vi "save_mpi_hdf.vi"(3 "System Information cluster":T1, 5 "Subject metadata cluster":T2, 7 "Device Name":tag="DAQ2", 8 "TxRxParams":T3={"sample rate"=1000000.0, "Transmit frequency"=25000.0, "Transmit amplitude"=1.577, "sample rate digital out"=40000.0, "TX cycles"=600, "sample rate DAQ1"=1000000.0, "Receive frequency"=75000.0, "Receive range"=1.0, "TX harmonics"=[50000.0, 75000.0, 100000.0, 125000.0, 150000.0, 175000.0, 200000.0, 225000.0]} {"TX harmonics" format="%#_6p"; "Receive frequency" format="%#_6p"; "sample rate DAQ1" format="%#_6p"; "sample rate digital out" format="%#_6p"; "Transmit frequency" format="%#_6p"; "sample rate" format="%#_6p"}, 9 "image dataset":string, 10 "Path":path, 11 "Cluster in":T4={"Magnitude meas."=[], "Phase meas."=[], "Shift meas."=[], "cw"=TRUE, "projections per image"=0, "ramp-up readouts"=0, "current sense type"="", "Number of pulses per image"=0, "Rotation enabled"=TRUE, "Rotary position"=[], "Baseline magnitude"=0.0, "Baseline phase"=0.0, "Wait readouts"=0, "Shift waveform type"="", "Shift enabled"=TRUE, "Time domain data"=[], "Motor pulse duration"=0.0, "Shift Amp pk"=0.0, "Shift DC offset"=0.0, "Notes"="", "Reconstructed image"=bytes[0], "Rotary encoder type"="", "Image start"=timestamp(0 s since 1904-01-01), "Image stop"=timestamp(0 s since 1904-01-01), "readouts per projection"=0, "Recon enabled"=FALSE, "Bidirectional shift"=FALSE, "Imager mode"="", "Shift delay"=0.0, "Shift frequency"=0.0, "Image time (calc)"=0.0, "Initial encoder position"=0.0, "Recon data"=[], "Trigger line values"=[], "Bed position"=0.0, "Sample image"=bytes[0], "Patch amplitude"=0.0, "Patch frequency"=0.0, "Patch phase"=0.0, "proj mag f2-f9"=[], "proj phase f2-f9"=[], "Tx waveform"=[], "Tx FFT mag"=[], "Tx FFT phase"=[], "Temps"=[]}) -> ()   [LabVIEW 2021]
uses:
  <vilib>/UPVI/lvhdf5/file.llb/LVH5F Operation.ctl
  <vilib>/Utility/miscctls.llb/LVRectTypeDef.ctl
  <vilib>/UPVI/lvhdf5/group.llb/H5G_obj_t.ctl
  <vilib>/UPVI/lvhdf5/dataset.llb/LVH5D Operation.ctl
  <vilib>/UPVI/lvhdf5/attribute.llb/LVH5A Operation.ctl
  <vilib>/UPVI/lvhdf5/identifier.llb/Not an HDF5 Refnum Constant.vi
  <vilib>/UPVI/lvhdf5/utility.llb/Select HDF5 Dialog.vi
  <vilib>/UPVI/lvhdf5/utility.llb/Select HDF5 Dialog (Object Only).vi
  <vilib>/UPVI/lvhdf5/dataset.llb/Simple H5Dwrite (Variant).vi
  <vilib>/UPVI/lvhdf5/common.llb/To HDF5 Ref.vi
  <vilib>/UPVI/lvhdf5/dataset.llb/H5Dclose.vi
  <vilib>/UPVI/lvhdf5/attribute.llb/LVH5 Write Attributes.xnode
  <vilib>/UPVI/lvhdf5/library.llb/HDF5 Ref.ctl
  <vilib>/UPVI/lvhdf5/dataset.llb/Simple H5Dwrite.xnode
  <vilib>/UPVI/lvhdf5/dataset.llb/Write Dataset with Attributes.xnode
  <vilib>/UPVI/lvhdf5/attribute.llb/Cluster to Attribute Array.xnode
  <vilib>/Utility/error.llb/Error Cluster From Error Code.vi
  <vilib>/UPVI/lvhdf5/dataset.llb/OpenCreateReplace Dataset by Element Type.vi
  <vilib>/UPVI/lvhdf5/dataspace.llb/H5Sselect_hyperslab.vi
  <vilib>/UPVI/lvhdf5/dataset.llb/H5Dwrite (Variant).vi
  <vilib>/UPVI/lvhdf5/dataset.llb/H5Dget_space.vi
  <vilib>/UPVI/lvhdf5/attribute.llb/private/LVH5AwriteWDTAttrs.vi
  <vilib>/UPVI/lvhdf5/dataspace.llb/H5Sclose.vi
  <vilib>/UPVI/lvhdf5/utility.llb/Select HDF5 Dialog (File and Object).vi
  <resource>/objmgr/daqmx.rc
  <vilib>/UPVI/lvhdf5/library.llb/HDF5 Ref.lvclass
  <vilib>/Utility/Data Type/Get Type Information.vi
  <vilib>/Utility/Data Type/NI_Data Type.lvlib
  <vilib>/Utility/Data Type/Get Cluster Information.vi
panel:
  in  "OnlineReconPath":path
  out "appended path":path
  out "error out":errorcluster
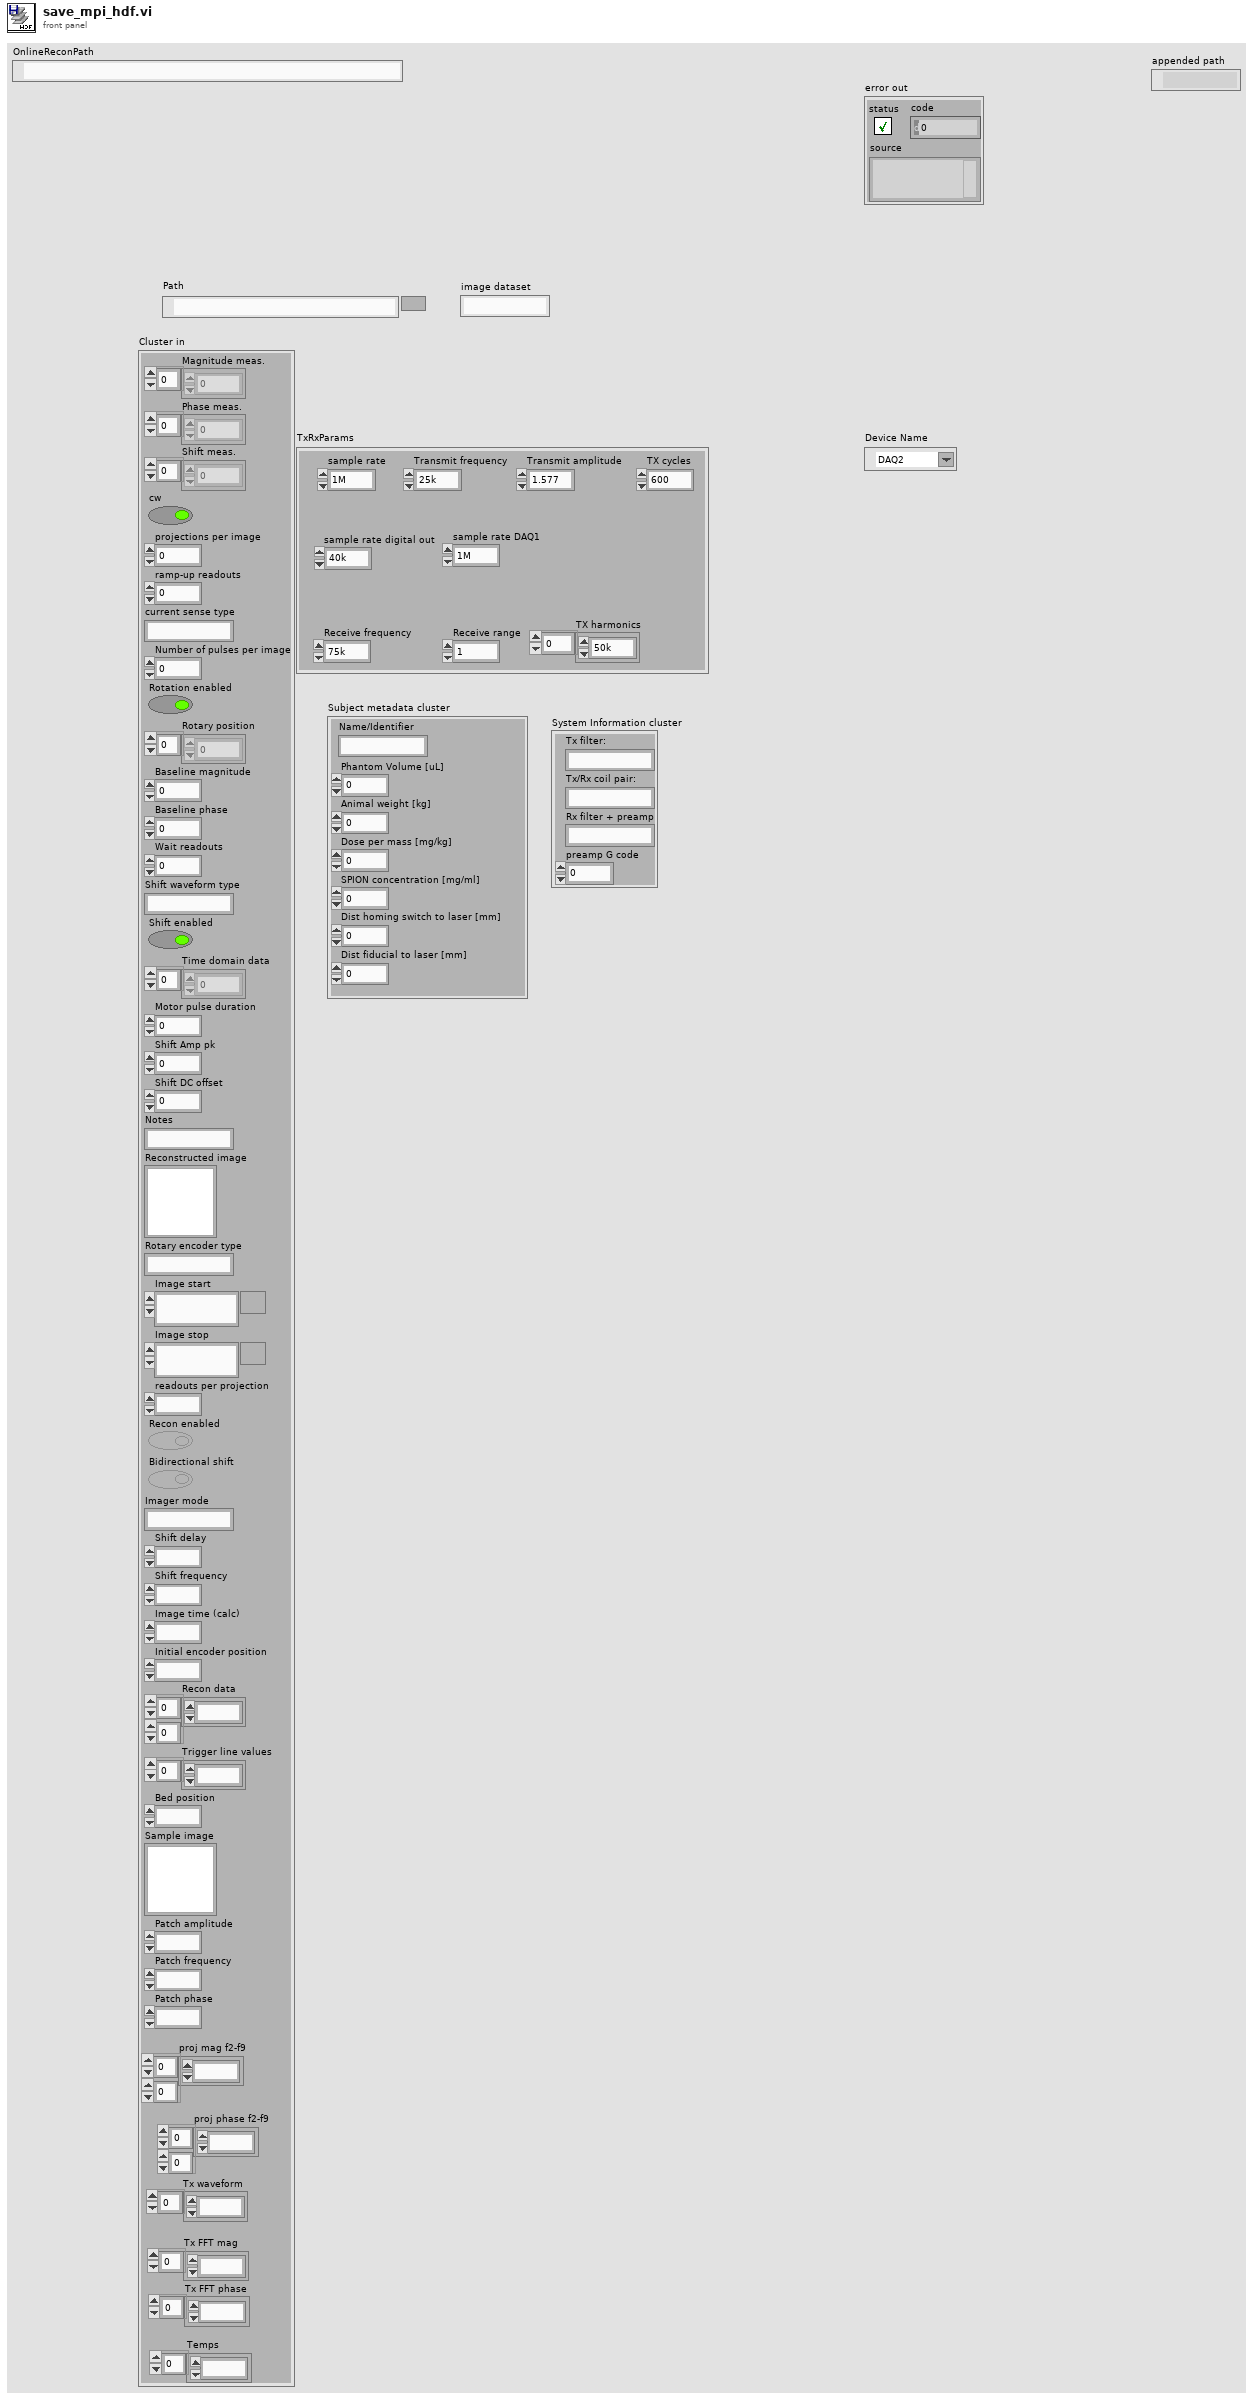
[diagram p1: front panel]
types:
  T1 = cluster{"Tx filter:":string, "Tx/Rx coil pair:":string, "Rx filter + preamp":string, "preamp G code":dbl}
  T2 = cluster{"Name/Identifier":string, "Phantom Volume [uL]":dbl, "Animal weight [kg]":dbl, "Dose per mass [mg/kg]":dbl, "SPION concentration [mg/ml]":dbl, "Dist homing switch to laser [mm]":dbl, "Dist fiducial to laser [mm]":dbl}
  T3 = cluster{"sample rate":dbl, "Transmit frequency":dbl, "Transmit amplitude":dbl, "sample rate digital out":dbl, "TX cycles":i32, "sample rate DAQ1":dbl, "Receive frequency":dbl, "Receive range":dbl, "TX harmonics":dbl[]}
  T4 = cluster{"Magnitude meas.":dbl[], "Phase meas.":dbl[], "Shift meas.":dbl[], "cw":bool, "projections per image":i32, "ramp-up readouts":i32, "current sense type":string, "Number of pulses per image":i32, "Rotation enabled":bool, "Rotary position":dbl[], "Baseline magnitude":dbl, "Baseline phase":dbl, "Wait readouts":i32, "Shift waveform type":string, "Shift enabled":bool, "Time domain data":dbl[], "Motor pulse duration":dbl, "Shift Amp pk":dbl, "Shift DC offset":dbl, "Notes":string, "Reconstructed image":picture, "Rotary encoder type":string, "Image start":timestamp, "Image stop":timestamp, "readouts per projection":i32, "Recon enabled":bool, "Bidirectional shift":bool, "Imager mode":string, "Shift delay":dbl, "Shift frequency":dbl, "Image time (calc)":dbl, "Initial encoder position":dbl, "Recon data":dbl[][], "Trigger line values":i32[], "Bed position":dbl, "Sample image":picture, "Patch amplitude":dbl, "Patch frequency":dbl, "Patch phase":dbl, "proj mag f2-f9":dbl[][], "proj phase f2-f9":dbl[][], "Tx waveform":dbl[], "Tx FFT mag":dbl[], "Tx FFT phase":dbl[], "Temps":dbl[]}
  T5 = typedef "LVH5F Operation.ctl" = enum16{"open", "open or create", "create or replace", "create or replace (with confirmation)", "create", "open (read only)"}
  T6 = typedef "HDF5 Ref.ctl" = refnum<class "HDF5 Ref.lvclass">
  T7 = typedef "LVRectTypeDef.ctl" = cluster{"Left":i16, "Top":i16, "Right":i16, "Bottom":i16}
  T8 = cluster{"Behavior":enum32{"Invalid", "Default", "Floating", "Floating/Auto-Hide", "Modal"}, "Position":T7, "Center":bool, "Title":string}
  T9 = typedef "LVH5D Operation.ctl" = enum16{"open", "replace", "create", "open or create", "create or replace", "create or replace with confirmation"}
  T10 = typedef "H5G_obj_t.ctl" = i32
  T11 = cluster{"Object Types (any)":T10[], "Object Pattern":string}
  T12 = typedef "LVH5A Operation.ctl" = enum16{"open", "replace", "create", "open or create", "create or replace", "create or replace with confirmation"}
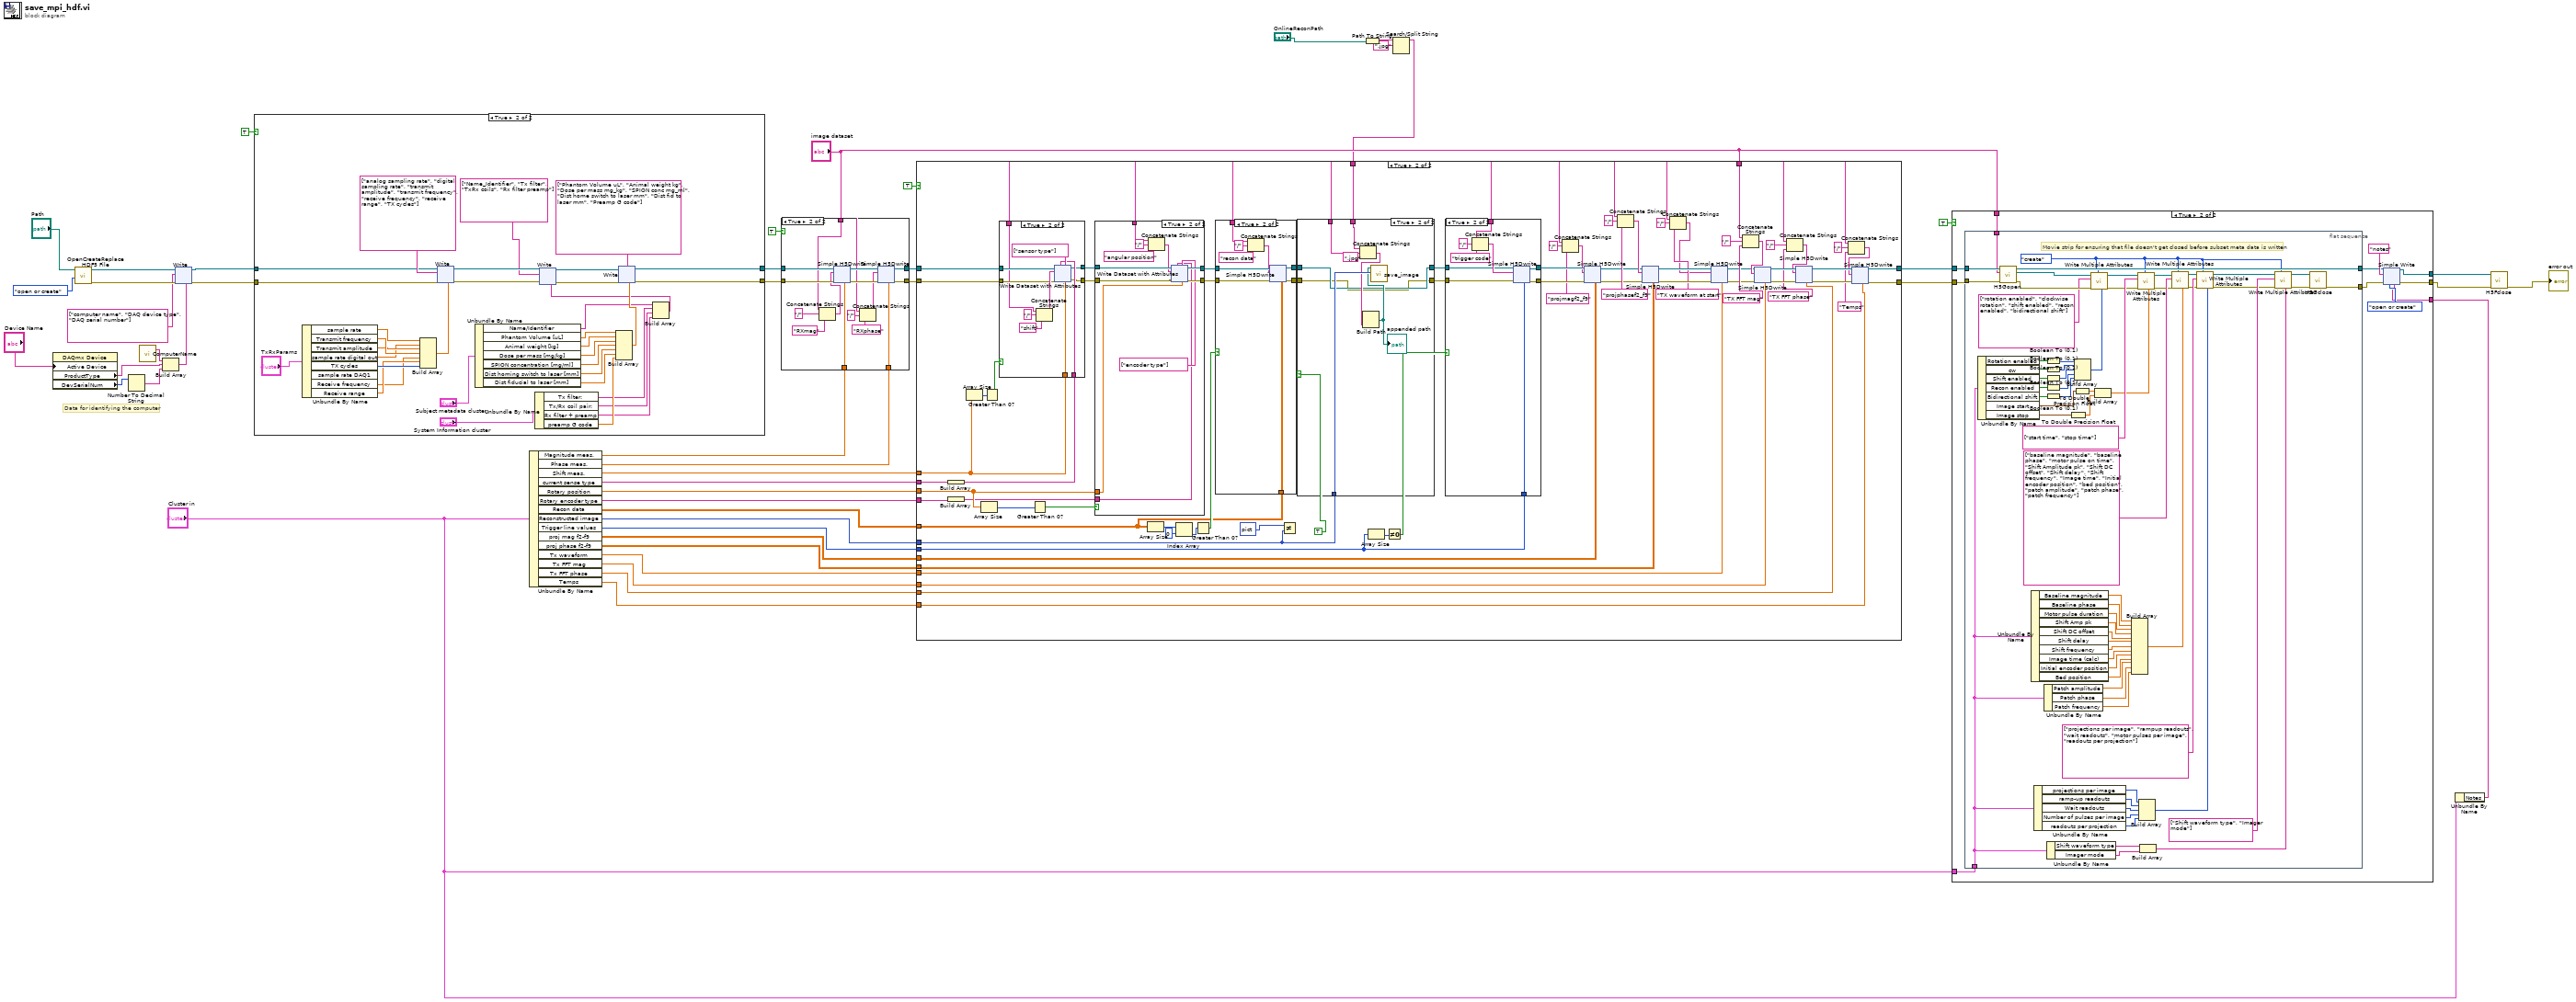
[diagram p0: block diagram]
diagram:
  # "Data for identifying the computer"
  n1 = property class="DAQmx Device"("Active Device"="Device Name") -> ("ProductType"=w11:string, "DevSerialNum"=w9:u32)  [unwired: 2 in, 2 out]
  n2 = call <vilib>:"OpenCreateReplace HDF5 File.vi"("function (open or create)"=LVH5F_Operation."open or create", "path"="Path") -> ("error out"=w46:errorcluster, "HDF5 Ref out"=w47:T6)  [unwired: 6 in]
  n3 = Number To Decimal String(number=w9) -> (decimal integer string=w10:string)  [unwired: 1 in]
  n4 = call "ComputerName.vi"() -> ("String/Binary data"=w12:string)  [unwired: 4 in, 1 out]
  n5 = Build Array(w12, w11, w10) -> (w13:string[])
  n6 = xnode "Write"("HDF5 Ref"=w47, "error in (no error)"=w46, "Name(s)"=string[] ["computer name", "DAQ device type", "DAQ serial number"], "Value(s)"=w13) -> ("HDF5 Ref out"=w7:T6, "error out"=w6:errorcluster)  [unwired: 1 in]
  n7 = case shown="True" TRUE {
    tunnel: [w50 w71] -> w45
    tunnel: [w49 w68] -> w44
    tunnel: w7 -> [w50 w84]
    tunnel: w6 -> [w49 w83]
    frame False {
    }
    frame True {
      n8 = Unbundle By Name("TxRxParams") -> ("sample rate"=w75:dbl, "Transmit frequency"=w78:dbl, "Transmit amplitude"=w77:dbl, "sample rate digital out"=w76:dbl, "TX cycles"=w81:i32, "Receive frequency"=w79:dbl, "Receive range"=w80:dbl)  [unwired: 1 out]
      n9 = Build Array(w75, w76, w77, w78, w79, w80, w81) -> (w74:dbl[])
      n10 = xnode "Write"("HDF5 Ref"=w84, "error in (no error)"=w83, "Name(s)"=string[] ["analog sampling rate", "digital sampling rate", "transmit amplitude", "transmit frequency", "receive frequency", "receive range", "TX cycles"], "Value(s)"=w74) -> ("HDF5 Ref out"=w73:T6, "error out"=w70:errorcluster)  [unwired: 1 in]
      n11 = Unbundle By Name("Subject metadata cluster") -> ("Name/Identifier"=w57:string, "Phantom Volume [uL]"=w64:dbl, "Animal weight [kg]"=w63:dbl, "Dose per mass [mg/kg]"=w62:dbl, "SPION concentration [mg/ml]"=w61:dbl, "Dist homing switch to laser [mm]"=w60:dbl, "Dist fiducial to laser [mm]"=w59:dbl)
      n12 = Unbundle By Name("System Information cluster") -> ("Tx filter:"=w54:string, "Tx/Rx coil pair:"=w53:string, "Rx filter + preamp"=w52:string, "preamp G code"=w55:dbl)
      n13 = Build Array(w64, w63, w62, w61, w60, w59, w55) -> (w65:dbl[])
      n14 = Build Array(w57, w54, w53, w52) -> (w58:string[])
      n15 = xnode "Write"("HDF5 Ref"=w73, "error in (no error)"=w70, "Name(s)"=string[] ["Name_Identifier", "Tx filter", "TxRx coils", "Rx filter preamp"], "Value(s)"=w58) -> ("HDF5 Ref out"=w72:T6, "error out"=w69:errorcluster)  [unwired: 1 in]
      n16 = xnode "Write"("HDF5 Ref"=w72, "error in (no error)"=w69, "Name(s)"=string[] ["Phantom Volume uL", "Animal weight kg", "Dose per mass mg_kg", "SPION conc mg_ml", "Dist home switch to laser mm", "Dist fid to laser mm", "Preamp G code"], "Value(s)"=w65) -> ("HDF5 Ref out"=w71:T6, "error out"=w68:errorcluster)  [unwired: 1 in]
    }
  }
  n17 = Unbundle By Name("Cluster in") -> ("Magnitude meas."=w33:dbl[], "Phase meas."=w43:dbl[], "Shift meas."=w37:dbl[], "current sense type"=w40:string, "Rotary position"=w38:dbl[], "Rotary encoder type"=w39:string, "Recon data"=w32:dbl[][], "Reconstructed image"=w36:picture, "Trigger line values"=w35:i32[], "proj mag f2-f9"=w31:dbl[][], "proj phase f2-f9"=w30:dbl[][], "Tx waveform"=w29:dbl[], "Tx FFT mag"=w28:dbl[], "Tx FFT phase"=w27:dbl[], "Temps"=w23:dbl[])
  n18 = case shown="True" TRUE {
    tunnel: w45 -> [w429 w442]
    tunnel: w44 -> [w428 w441]
    tunnel: w43 -> [_ w434]
    tunnel: [w429 w433] -> w42
    tunnel: [w428 w432] -> w41
    tunnel: w33 -> [_ w431]
    tunnel: "image dataset" -> [_ w430]
    frame False {
    }
    frame True {
      n19 = Concatenate Strings(w430, "/" ("string"), "RXmag" ("string")) -> (w440:string)
      n20 = xnode "Simple H5Dwrite"("Dataset Path"=w440, "error in (no error)"=w441, "HDF5 Path or Ref"=w442, "Data"=w431) -> ("HDF5 Ref out"=w439:T6, "error out"=w438:errorcluster)  [unwired: 4 in, 1 out]
      n21 = Concatenate Strings(w430, "/" ("string"), "RXphase" ("string")) -> (w435:string)
      n22 = xnode "Simple H5Dwrite"("Dataset Path"=w435, "error in (no error)"=w438, "HDF5 Path or Ref"=w439, "Data"=w434) -> ("HDF5 Ref out"=w433:T6, "error out"=w432:errorcluster)  [unwired: 4 in, 1 out]
    }
  }
  n23 = Path To String(path="OnlineReconPath") -> (string=w5:string)
  n24 = Search/Split String(string=w5, search string/char (-)=".jpg") -> (substring before match=w2:string)  [unwired: 1 in, 2 out]
  n25 = case shown="True" TRUE {
    tunnel: w42 -> [w850 w921]
    tunnel: w41 -> [w849 w920]
    tunnel: w40 -> [_ w919]
    tunnel: w39 -> [_ w917]
    tunnel: w38 -> [_ w914]
    tunnel: w37 -> [_ w908]
    tunnel: w36 -> [_ w902]
    tunnel: w35 -> [_ w894]
    tunnel: w32 -> [_ w887]
    tunnel: w31 -> [_ w886]
    tunnel: w30 -> [_ w880]
    tunnel: w29 -> [_ w874]
    tunnel: w28 -> [_ w863]
    tunnel: w27 -> [_ w862]
    tunnel: [w850 w860] -> w26
    tunnel: [w849 w858] -> w25
    tunnel: "image dataset" -> [_ w856]
    tunnel: w23 -> [_ w854]
    tunnel: w2 -> [_ w851]
    frame False {
    }
    frame True {
      n26 = Build Array(w919) -> (w918:string[])
      n27 = Build Array(w917) -> (w911:string[])
      n28 = Array Size(array=w908) -> (size(s)=w909:i32)
      n29 = Array Size(array=w914) -> (size(s)=w913:i32)
      n30 = Greater Than 0?(x=w909) -> (x > 0?=w910:bool)
      n31 = case shown="True" w910 {
        tunnel: w921 -> [w2571 w2579]
        tunnel: w920 -> [w2570 w2578]
        tunnel: w908 -> [_ w2577]
        tunnel: w918 -> [_ w2575]
        tunnel: [w2571 w2574] -> w916
        tunnel: [w2570 w2573] -> w915
        tunnel: w856 -> [_ w2572]
        frame False {
        }
        frame True {
          n32 = Concatenate Strings(w2572, "/" ("string"), "shift" ("string")) -> (w2582:string)
          n33 = xnode "Write Dataset with Attributes"("Dataset Path"=w2582, "error in (no error)"=w2578, "HDF5 Path or Ref"=w2579, "Attribute Name(s)"=string[] ["sensor type"], "Attribute Value(s)"=w2575, "Data"=w2577) -> ("HDF5 Ref out"=w2574:T6, "error out"=w2573:errorcluster)  [unwired: 2 in, 1 out]
        }
      }
      n34 = Greater Than 0?(x=w913) -> (x > 0?=w912:bool)
      n35 = case shown="True" w912 {
        tunnel: w916 -> [w2878 w2886]
        tunnel: w915 -> [w2877 w2885]
        tunnel: [w2878 w2884] -> w907
        tunnel: [w2877 w2883] -> w906
        tunnel: w914 -> [_ w2880]
        tunnel: w856 -> [_ w2887]
        tunnel: w911 -> [_ w2879]
        frame False {
        }
        frame True {
          n36 = Concatenate Strings(w2887, "/" ("string"), "angular position" ("string")) -> (w2881:string)
          n37 = xnode "Write Dataset with Attributes"("Dataset Path"=w2881, "error in (no error)"=w2885, "HDF5 Path or Ref"=w2886, "Attribute Name(s)"=string[] ["encoder type"], "Attribute Value(s)"=w2879, "Data"=w2880) -> ("HDF5 Ref out"=w2884:T6, "error out"=w2883:errorcluster)  [unwired: 2 in, 1 out]
        }
      }
      n38 = Array Size(array=w887) -> (size(s)=w901:i32[])
      n39 = Index Array(array=w901, index=0) -> (element=w899:i32)
      n40 = Greater Than 0?(x=w899) -> (x > 0?=w891:bool)
      n41 = case shown="True" w891 {
        tunnel: [w2358 w2367] -> w905
        tunnel: [w2357 w2366] -> w904
        tunnel: w907 -> [w2358 w2365]
        tunnel: w906 -> [w2357 w2364]
        tunnel: w856 -> [_ w2360]
        tunnel: w887 -> [_ w2359]
        frame False {
        }
        frame True {
          n42 = Concatenate Strings(w2360, "/" ("string"), "recon data" ("string")) -> (w2361:string)
          n43 = xnode "Simple H5Dwrite"("Dataset Path"=w2361, "error in (no error)"=w2364, "HDF5 Path or Ref"=w2365, "Data"=w2359) -> ("HDF5 Ref out"=w2367:T6, "error out"=w2366:errorcluster)  [unwired: 4 in, 1 out]
        }
      }
      n44 = Not Equal?(x=picture data[5B] ("Reconstructed image"), y=w902) -> ()  [unwired: 1 out]
      n45 = case shown="True" TRUE {
        tunnel: w905 -> [w2348 w2351]
        tunnel: [w2348 w2351] -> w898
        tunnel: [w2347 w2350] -> w897
        tunnel: w904 -> [w2347 w2350]
        tunnel: w902 -> [_ w2356]
        tunnel: w856 -> [_ w2355]
        tunnel: w851 -> [_ w2349]
        frame False {
        }
        frame True {
          n46 = Concatenate Strings(w2349, w2355, ".jpg" ("string")) -> (w2353:string)
          n47 = Build Path(name or relative path=w2353) -> (appended path=w2352:path)  [unwired: 1 in]
          "appended path" <- w2352
          n48 = call "save_image.vi"("picture"=w2356, "path to JPEG file"=w2352) -> ()  [unwired: 10 in]
        }
      }
      n49 = Array Size(array=w894) -> (size(s)=w896:i32)
      n50 = Not Equal To 0?(x=w896) -> (x != 0?=w895:bool)
      n51 = case shown="True" w895 {
        tunnel: w898 -> [w2135 w2140]
        tunnel: w897 -> [w2134 w2141]
        tunnel: [w2135 w2139] -> w892
        tunnel: [w2134 w2138] -> w893
        tunnel: w856 -> [_ w2137]
        tunnel: w894 -> [_ w2136]
        frame False {
        }
        frame True {
          n52 = Concatenate Strings(w2137, "/" ("string"), "trigger code" ("string")) -> (w2142:string)
          n53 = xnode "Simple H5Dwrite"("Dataset Path"=w2142, "error in (no error)"=w2141, "HDF5 Path or Ref"=w2140, "Data"=w2136) -> ("HDF5 Ref out"=w2139:T6, "error out"=w2138:errorcluster)  [unwired: 4 in, 1 out]
        }
      }
      n54 = Concatenate Strings(w856, "/" ("string"), "projmagf2_f9" ("string")) -> (w888:string)
      n55 = xnode "Simple H5Dwrite"("Dataset Path"=w888, "error in (no error)"=w893, "HDF5 Path or Ref"=w892, "Data"=w886) -> ("HDF5 Ref out"=w882:T6, "error out"=w881:errorcluster)  [unwired: 4 in, 1 out]
      n56 = Concatenate Strings(w856, "/" ("string"), "projphasef2_f9" ("string")) -> (w885:string)
      n57 = xnode "Simple H5Dwrite"("Dataset Path"=w885, "error in (no error)"=w881, "HDF5 Path or Ref"=w882, "Data"=w880) -> ("HDF5 Ref out"=w879:T6, "error out"=w878:errorcluster)  [unwired: 4 in, 1 out]
      n58 = Concatenate Strings(w856, "/" ("string"), "TX waveform at start" ("string")) -> (w875:string)
      n59 = xnode "Simple H5Dwrite"("Dataset Path"=w875, "error in (no error)"=w878, "HDF5 Path or Ref"=w879, "Data"=w874) -> ("HDF5 Ref out"=w865:T6, "error out"=w864:errorcluster)  [unwired: 4 in, 1 out]
      n60 = Concatenate Strings(w856, "/" ("string"), "TX FFT mag" ("string")) -> (w869:string)
      n61 = xnode "Simple H5Dwrite"("Dataset Path"=w869, "error in (no error)"=w864, "HDF5 Path or Ref"=w865, "Data"=w863) -> ("HDF5 Ref out"=w872:T6, "error out"=w873:errorcluster)  [unwired: 4 in, 1 out]
      n62 = Concatenate Strings(w856, "/" ("string"), "TX FFT phase" ("string")) -> (w866:string)
      n63 = xnode "Simple H5Dwrite"("Dataset Path"=w866, "error in (no error)"=w873, "HDF5 Path or Ref"=w872, "Data"=w862) -> ("HDF5 Ref out"=w861:T6, "error out"=w859:errorcluster)  [unwired: 4 in, 1 out]
      n64 = Concatenate Strings(w856, "/" ("string"), "Temps" ("string")) -> (w853:string)
      n65 = xnode "Simple H5Dwrite"("Dataset Path"=w853, "error in (no error)"=w859, "HDF5 Path or Ref"=w861, "Data"=w854) -> ("HDF5 Ref out"=w860:T6, "error out"=w858:errorcluster)  [unwired: 4 in, 1 out]
    }
  }
  n66 = Unbundle By Name("Cluster in") -> ("Notes"=w20:string)
  n67 = case shown="True" TRUE {
    tunnel: "Cluster in" -> [_ w3196]
    tunnel: w26 -> [w3184 w3195]
    tunnel: w25 -> [w3185 w3194]
    tunnel: "image dataset" -> [_ w3193]
    tunnel: w20 -> [_ w3188]
    tunnel: [w3184 w3187] -> w19
    tunnel: [w3185 w3186] -> w18
    frame False {
    }
    frame True {
      n68 = flat-sequence {
        tunnel: w3194 -> [w3454]
        tunnel: w3195 -> [w3461]
        tunnel: w3196 -> [w3407]
        tunnel: w3193 -> [w3460]
        tunnel: [w3399] -> w3191
        tunnel: [w3438] -> w3189
        frame #0 {
          w3402 = LVH5A_Operation."create" ("operation (open or create)")
          # "Movie strip for ensuring that file doesn't get closed before subset meta data is written"
          n69 = Unbundle By Name(w3407) -> ("Rotation enabled"=w3417:bool, "cw"=w3414:bool, "Shift enabled"=w3413:bool, "Recon enabled"=w3411:bool, "Bidirectional shift"=w3409:bool, "Image start"=w3453:timestamp, "Image stop"=w3450:timestamp)
          n70 = call <vilib>:"H5Gopen.vi"("error in (no error)"=w3454, "Name"=w3460, "HDF5 Ref"=w3461) -> ("error out"=w3420:errorcluster, "HDF5 Group Ref"=w3423:T6, "HDF5 Ref out"=w3438:T6)  [unwired: 4 in]
          n71 = Unbundle By Name(w3407) -> ("Baseline magnitude"=w3459:dbl, "Baseline phase"=w3458:dbl, "Motor pulse duration"=w3457:dbl, "Shift Amp pk"=w3456:dbl, "Shift DC offset"=w3455:dbl, "Shift delay"=w3443:dbl, "Shift frequency"=w3442:dbl, "Image time (calc)"=w3441:dbl, "Initial encoder position"=w3439:dbl, "Bed position"=w3403:dbl)
          n72 = Unbundle By Name(w3407) -> ("projections per image"=w3449:i32, "ramp-up readouts"=w3448:i32, "Wait readouts"=w3447:i32, "Number of pulses per image"=w3446:i32, "readouts per projection"=w3444:i32)
          n73 = Unbundle By Name(w3407) -> ("Patch amplitude"=w3404:dbl, "Patch phase"=w3405:dbl, "Patch frequency"=w3406:dbl)
          n74 = Boolean To (0,1)(Boolean=w3417) -> (0, 1=w3416:i16)
          n75 = Boolean To (0,1)(Boolean=w3414) -> (0, 1=w3415:i16)
          n76 = Boolean To (0,1)(Boolean=w3413) -> (0, 1=w3412:i16)
          n77 = Boolean To (0,1)(Boolean=w3411) -> (0, 1=w3410:i16)
          n78 = Boolean To (0,1)(Boolean=w3409) -> (0, 1=w3408:i16)
          n79 = Unbundle By Name(w3407) -> ("Shift waveform type"=w3445:string, "Imager mode"=w3440:string)
          n80 = To Double Precision Float(number=w3450) -> (double precision float=w3451:dbl)
          n81 = Build Array(w3416, w3415, w3412, w3410, w3408) -> (w3418:i16[])
          n82 = To Double Precision Float(number=w3453) -> (double precision float=w3452:dbl)
          n83 = call <vilib>:"Write Multiple Attributes.vi"("Values"=w3418, "operation (open or create)"=w3402, "error in (no error)"=w3420, "Names"=string[] ["rotation enabled", "clockwise rotation", "shift enabled", "recon enabled", "bidirectional shift"] ("Name(s)"), "HDF5 Ref"=w3423) -> ("error out"=w3421:errorcluster, "HDF5 Ref out"=w3422:T6)  [unwired: 3 in]
          n84 = Build Array(w3452, w3451) -> (w3424:dbl[])
          n85 = Build Array(w3459, w3458, w3457, w3456, w3455, w3443, w3442, w3441, w3439, w3403, w3404, w3405, w3406) -> (w3428:dbl[])
          n86 = call <vilib>:"Write Multiple Attributes.vi"("Values"=w3424, "operation (open or create)"=w3402, "error in (no error)"=w3421, "Names"=string[] ["start time", "stop time"] ("Name(s)"), "HDF5 Ref"=w3422) -> ("error out"=w3426:errorcluster, "HDF5 Ref out"=w3427:T6)  [unwired: 3 in]
          n87 = Build Array(w3449, w3448, w3447, w3446, w3444) -> (w3432:i32[])
          n88 = Build Array(w3445, w3440) -> (w3436:string[])
          n89 = call <vilib>:"Write Multiple Attributes.vi"("Values"=w3428, "operation (open or create)"=w3402, "error in (no error)"=w3426, "Names"=string[] ["baseline magnitude", "baseline phase", "motor pulse on time", "Shift Amplitude pk", "Shift DC offset", "Shift delay", "Shift frequency", "Image time", "Initial encoder position", "bed position", "patch amplitude", "patch phase", "patch frequency"] ("Name(s)"), "HDF5 Ref"=w3427) -> ("error out"=w3430:errorcluster, "HDF5 Ref out"=w3431:T6)  [unwired: 3 in]
          n90 = call <vilib>:"Write Multiple Attributes.vi"("Values"=w3432, "operation (open or create)"=w3402, "error in (no error)"=w3430, "Names"=string[] ["projections per image", "rampup readouts", "wait readouts", "motor pulses per image", "readouts per projection"] ("Name(s)"), "HDF5 Ref"=w3431) -> ("error out"=w3433:errorcluster, "HDF5 Ref out"=w3435:T6)  [unwired: 3 in]
          n91 = call <vilib>:"Write Multiple Attributes.vi"("Values"=w3436, "operation (open or create)"=w3402, "error in (no error)"=w3433, "Names"=string[] ["Shift waveform type", "Imager mode"] ("Name(s)"), "HDF5 Ref"=w3435) -> ("error out"=w3400:errorcluster, "HDF5 Ref out"=w3401:T6)  [unwired: 3 in]
          n92 = call <vilib>:"H5Gclose.vi"("error in (no error)"=w3400, "HDF5 Group Ref"=w3401) -> ("error out"=w3399:errorcluster)  [unwired: 7 in]
        }
      }
      n93 = xnode "Simple Write"("Dataset Path"="notes", "error in (no error)"=w3191, "operation (open or create)"=LVH5D_Operation."open or create", "HDF5 Path or Ref"=w3189, "Data"=w3188) -> ("HDF5 Ref out"=w3187:T6, "error out"=w3186:errorcluster)  [unwired: 3 in, 1 out]
    }
  }
  n94 = call <vilib>:"H5Fclose.vi"("error in (no error)"=w18, "HDF5 Ref"=w19) -> ("error out"=→"error out":errorcluster)  [unwired: 7 in]
